vi "VisionNetwork.vi"(8 "error in (no error)":errorcluster) -> (0 "error out":errorcluster)   [LabVIEW 2023]
doc: "Vision Network\n\nInput\n --Error in \n\nOutput\n --Error out"
uses:
  <vilib>/Rock Robotics/WPI/ThirdParty/JAS_Junk/TrajLib/Rotation2d_CreateAngle.vi
  <vilib>/Rock Robotics/WPI/ThirdParty/JAS_Junk/TrajLib/Translation2d_Create.vi
  VisionGlobal.vi
  <vilib>/Rock Robotics/Network Tables/NT Write Number.vi
  <vilib>/Rock Robotics/Network Tables/NT Write Boolean.vi
  <vilib>/Rock Robotics/Network Tables/NT Read Number.vi
  <vilib>/Rock Robotics/WPI/ThirdParty/JAS_Junk/TrajLib/Trajectory_Library.lvlib
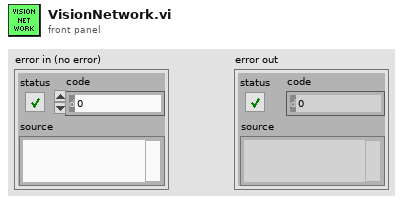
[diagram p1: front panel]
types:
  T1 = typedef "Trajectory_Library.lvlib/POSE2D.ctl" = cluster{"TRANSLATION":T2, "ROTATION":T3}
  T2 = typedef "Trajectory_Library.lvlib/TRANSLATION2D.ctl" = cluster{"X":dbl, "Y":dbl}
  T3 = typedef "Trajectory_Library.lvlib/ROTATION2D.ctl" = cluster{"VALUE":dbl, "COS":dbl, "SIN":dbl}
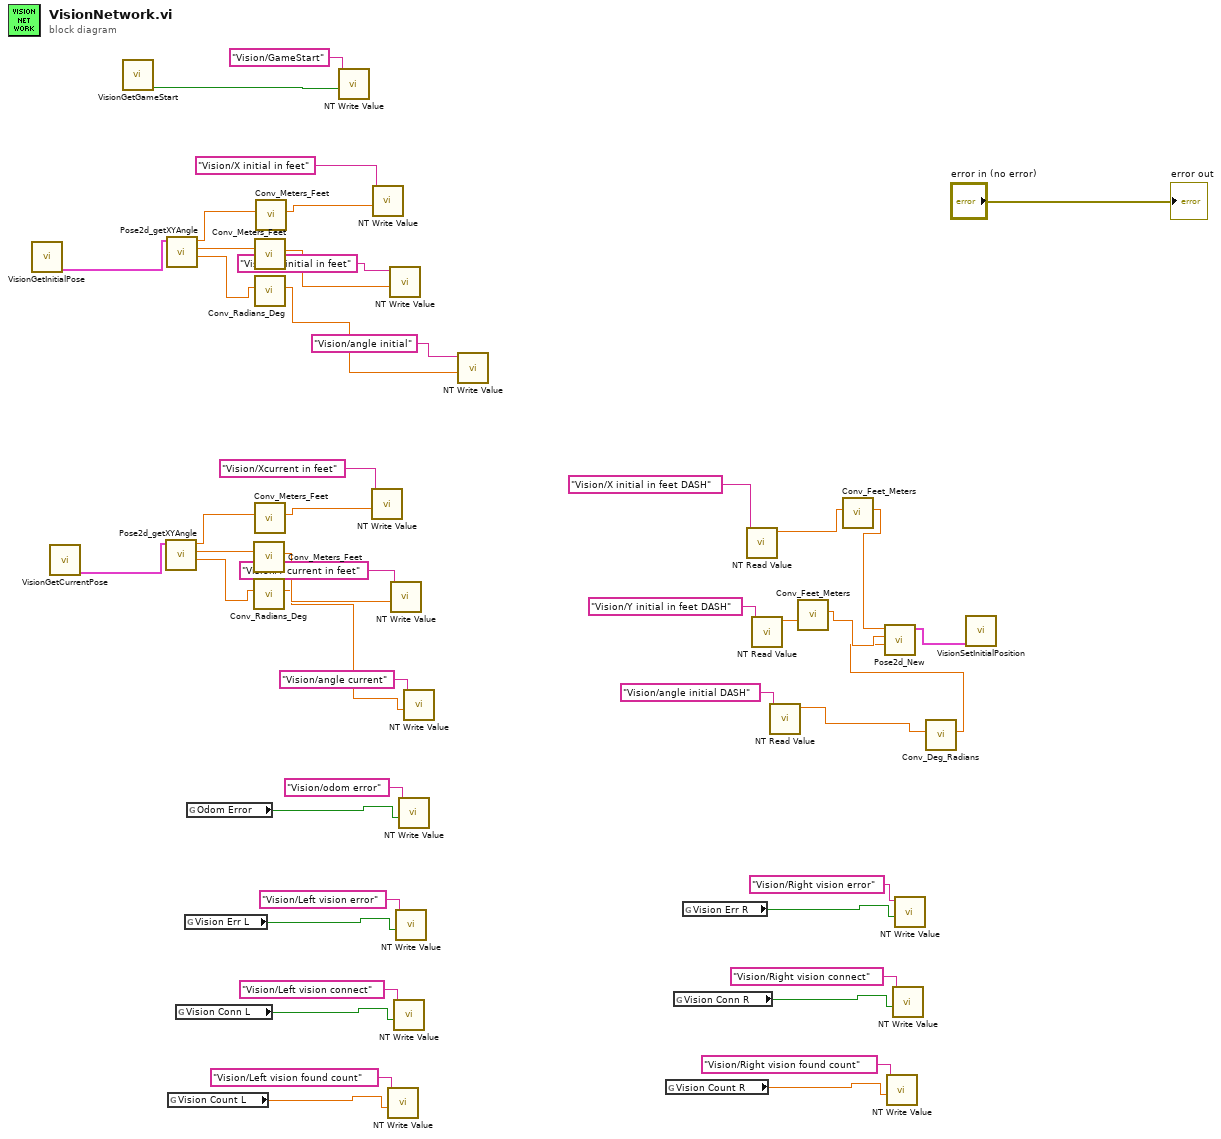
[diagram p0: block diagram]
diagram:
  n1 = call "VisionGetInitialPose.vi"() -> ("InitialPose"=w33:T1)  [unwired: 10 in]
  n2 = call "VisionGetCurrentPose.vi"() -> ("Current Pose"=w46:T1)  [unwired: 9 in]
  n3 = call "VisionGetGameStart.vi"() -> ("Game Start"=w32:bool)  [unwired: 11 in]
  n4 = call <vilib>:"Pose2d_getXYAngle.vi"("in POSE"=w46) -> ("Angle"=w45:dbl, "Y"=w44:dbl, "X"=w43:dbl)  [unwired: 8 in]
  n5 = call <vilib>:"Pose2d_getXYAngle.vi"("in POSE"=w33) -> ("Angle"=w39:dbl, "Y"=w38:dbl, "X"=w37:dbl)  [unwired: 8 in]
  n6 = global read "VisionGlobal.vi" "Vision Count L"() -> (w7:dbl)
  n7 = global read "VisionGlobal.vi" "Vision Conn L"() -> (w9:bool)
  n8 = global read "VisionGlobal.vi" "Vision Err L"() -> (w11:bool)
  n9 = global read "VisionGlobal.vi" "Odom Error"() -> (w13:bool)
  n10 = call <vilib>:"Conv_Meters_Feet.vi"("Meters"=w44) -> ("Feet"=w41:dbl)  [unwired: 10 in]
  n11 = call <vilib>:"Conv_Radians_Deg.vi"("Radians"=w45) -> ("Degrees"=w40:dbl)  [unwired: 10 in]
  n12 = call <vilib>:"Conv_Meters_Feet.vi"("Meters"=w38) -> ("Feet"=w35:dbl)  [unwired: 10 in]
  n13 = call <vilib>:"Conv_Radians_Deg.vi"("Radians"=w39) -> ("Degrees"=w34:dbl)  [unwired: 10 in]
  n14 = call <vilib>:"Conv_Meters_Feet.vi"("Meters"=w43) -> ("Feet"=w42:dbl)  [unwired: 10 in]
  n15 = call <vilib>:"Conv_Meters_Feet.vi"("Meters"=w37) -> ("Feet"=w36:dbl)  [unwired: 10 in]
  n16 = call-poly <vilib>:"NT Write Value.vi"("value"=w32, "name"="Vision/GameStart") -> ()  [unwired: 9 in, 1 out]
  n17 = call-poly <vilib>:"NT Write Value.vi"("value"=w42, "name"="Vision/Xcurrent in feet") -> ()  [unwired: 9 in, 1 out]
  n18 = call-poly <vilib>:"NT Write Value.vi"("value"=w36, "name"="Vision/X initial in feet") -> ()  [unwired: 9 in, 1 out]
  n19 = call-poly <vilib>:"NT Write Value.vi"("value"=w7, "name"="Vision/Left vision found count") -> ()  [unwired: 9 in, 1 out]
  n20 = call-poly <vilib>:"NT Write Value.vi"("value"=w35, "name"="Vision/Y initial in feet") -> ()  [unwired: 9 in, 1 out]
  n21 = call-poly <vilib>:"NT Write Value.vi"("value"=w41, "name"="Vision/Y current in feet") -> ()  [unwired: 9 in, 1 out]
  n22 = call-poly <vilib>:"NT Write Value.vi"("value"=w9, "name"="Vision/Left vision connect") -> ()  [unwired: 9 in, 1 out]
  n23 = call-poly <vilib>:"NT Write Value.vi"("value"=w11, "name"="Vision/Left vision error") -> ()  [unwired: 9 in, 1 out]
  n24 = call-poly <vilib>:"NT Write Value.vi"("value"=w13, "name"="Vision/odom error") -> ()  [unwired: 9 in, 1 out]
  n25 = call-poly <vilib>:"NT Write Value.vi"("value"=w40, "name"="Vision/angle current") -> ()  [unwired: 9 in, 1 out]
  n26 = call-poly <vilib>:"NT Write Value.vi"("value"=w34, "name"="Vision/angle initial") -> ()  [unwired: 9 in, 1 out]
  n27 = global read "VisionGlobal.vi" "Vision Count R"() -> (w2:dbl)
  n28 = global read "VisionGlobal.vi" "Vision Conn R"() -> (w4:bool)
  n29 = global read "VisionGlobal.vi" "Vision Err R"() -> (w6:bool)
  n30 = call-poly <vilib>:"NT Read Value.vi"("name"="Vision/X initial in feet DASH") -> ("value"=w22:dbl)  [unwired: 8 in, 2 out]
  n31 = call-poly <vilib>:"NT Read Value.vi"("name"="Vision/Y initial in feet DASH") -> ("value"=w21:dbl)  [unwired: 8 in, 2 out]
  n32 = call-poly <vilib>:"NT Read Value.vi"("name"="Vision/angle initial DASH") -> ("value"=w19:dbl)  [unwired: 8 in, 2 out]
  n33 = call <vilib>:"Conv_Feet_Meters.vi"("Feet"=w21) -> ("Meters"=w20:dbl)  [unwired: 10 in]
  n34 = call <vilib>:"Conv_Feet_Meters.vi"("Feet"=w22) -> ("Meters"=w23:dbl)  [unwired: 10 in]
  n35 = call-poly <vilib>:"NT Write Value.vi"("value"=w2, "name"="Vision/Right vision found count") -> ()  [unwired: 9 in, 1 out]
  n36 = call-poly <vilib>:"NT Write Value.vi"("value"=w4, "name"="Vision/Right vision connect") -> ()  [unwired: 9 in, 1 out]
  n37 = call-poly <vilib>:"NT Write Value.vi"("value"=w6, "name"="Vision/Right vision error") -> ()  [unwired: 9 in, 1 out]
  n38 = call <vilib>:"Conv_Deg_Radians.vi"("Degress"=w19) -> ("Radians"=w18:dbl)  [unwired: 10 in]
  n39 = call <vilib>:"Pose2d_New.vi"("Heading"=w18, "Y"=w20, "X"=w23) -> ("out POSe"=w24:T1)  [unwired: 8 in]
  n40 = call "VisionSetInitialPosition.vi"("InitialPose"=w24) -> ()  [unwired: 11 in]
  "error out" <- "error in (no error)"
